vi "MeasLink Plugin Path.vi"(11 "error in (no error)":errorcluster) -> (0 "Measurement UI Lib":path, 1 "Run Service":path, 2 "Measurement UI":path, 3 "Instrumentstudio Folder":path, 4 "New Code Module":path, 5 "Set Default Value":path, 6 "Wrapper Path":path, 8 "Result Control":path, 10 "Input Controls":path, 12 "Library":path, 13 "Type Specialization":path, 14 "Logic VI Path":path, 15 "error out":errorcluster)   [LabVIEW 2021, in "Path Functions.lvlib"]
uses:
  Path Functions.lvlib
  Converter Reusables/Converter Reusables.lvlib
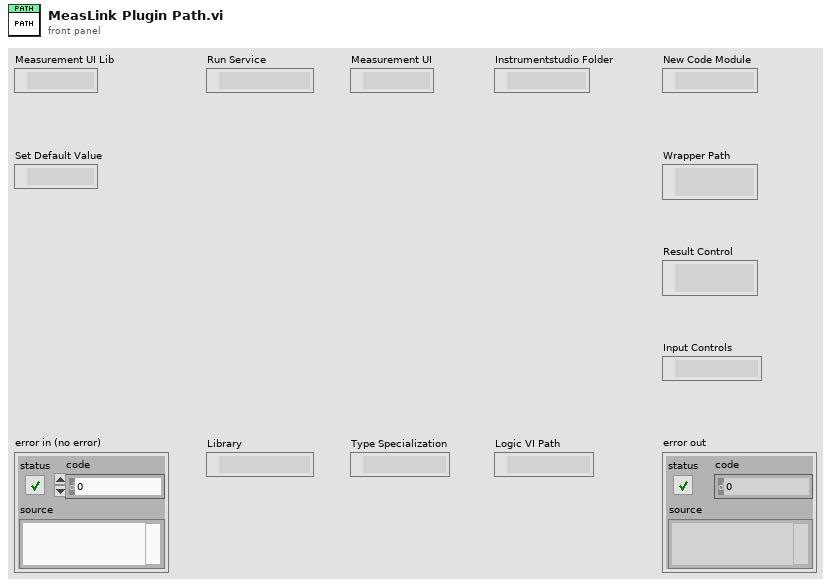
[diagram p1: front panel]
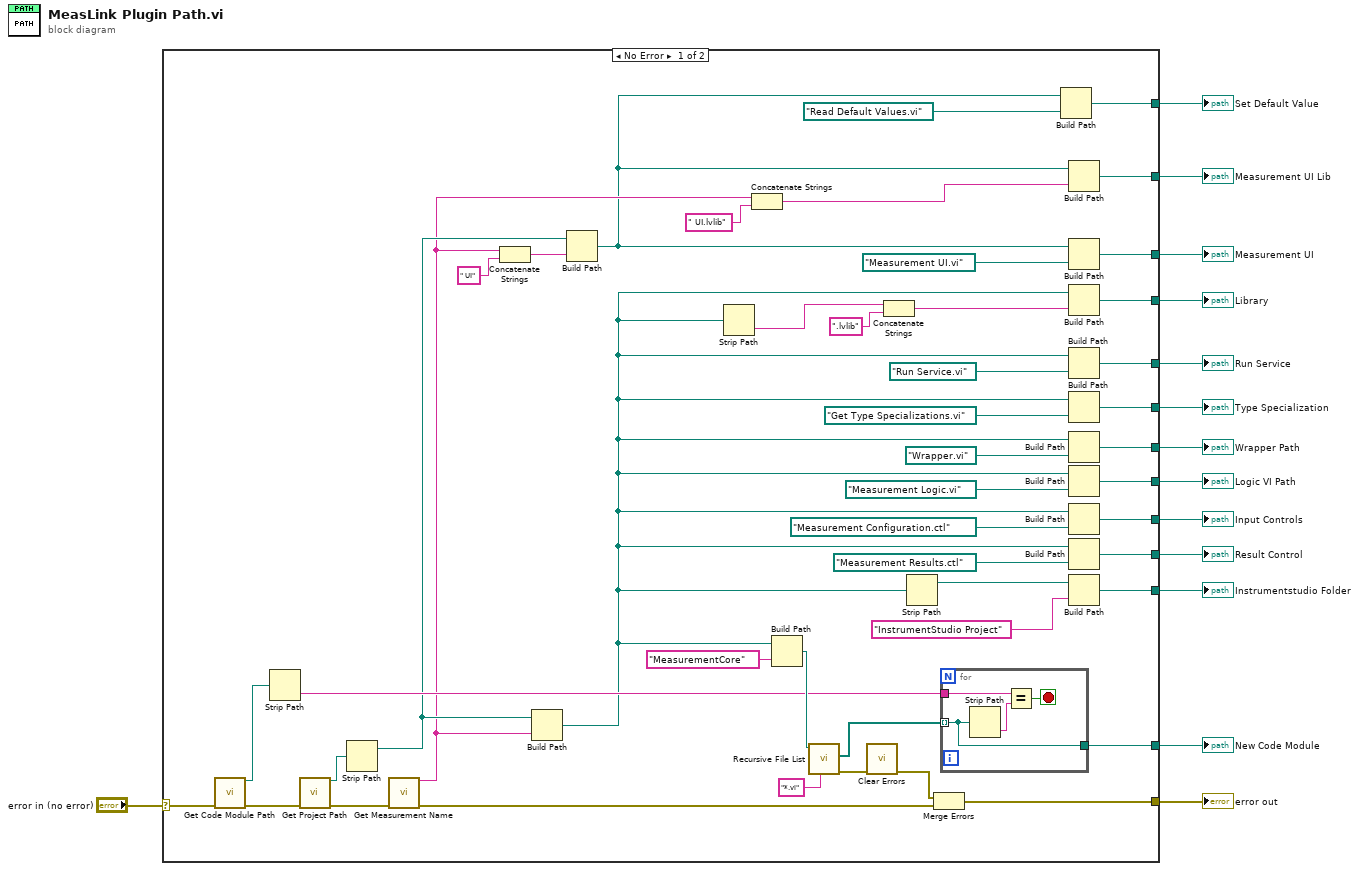
[diagram p0: block diagram]
diagram:
  n1 = case shown="No Error" "error in (no error)" {
    selector: "error in (no error)" -> [w42 w66]
    tunnel: [w61 _] -> w14
    tunnel: [w60 _] -> w13
    tunnel: [w59 _] -> w12
    tunnel: [w58 _] -> w11
    tunnel: [w52 _] -> w10
    tunnel: [w51 _] -> w9
    tunnel: [w49 _] -> w8
    tunnel: [w45 _] -> w7
    tunnel: [w38 _] -> w5
    tunnel: [w27 w66] -> w4
    tunnel: [w26 _] -> w3
    tunnel: [w18 _] -> w2
    tunnel: [w17 _] -> w1
    frame No Error {
      n2 = call "Get Code Module Path.vi"("error in (no error)"=w42) -> ("CodeModule Out"=w40:path, "error out"=w41:errorcluster)  [unwired: 13 in]
      n3 = Strip Path(path=w40) -> (name=w29:string)  [unwired: 1 out]
      n4 = call "Get Project Path.vi"("error in (no error)"=w41) -> ("Project Path Out"=w44:path, "error out"=w43:errorcluster)  [unwired: 13 in]
      n5 = Strip Path(path=w44) -> (stripped path=w24:path)  [unwired: 1 out]
      n6 = call "Get Measurement Name.vi"("error in (no error)"=w43) -> ("Name Out"=w19:string, "error out"=w28:errorcluster)  [unwired: 13 in]
      n7 = Concatenate Strings(w19, " UI" ("string")) -> (w22:string)
      n8 = Build Path(base path=w24, name or relative path=w19) -> (appended path=w25:path)
      n9 = Build Path(base path=w24, name or relative path=w22) -> (appended path=w16:path)
      n10 = Strip Path(path=w25) -> (name=w39:string)  [unwired: 1 out]
      n11 = Concatenate Strings(w19, " UI.lvlib" ("string")) -> (w20:string)
      n12 = Build Path(base path=w25, name or relative path="MeasurementCore" ("string")) -> (appended path=w32:path)
      n13 = call <vilib>:"Recursive File List.vi"("pattern"="*.vi", "Folder Path"=w32) -> ("error out"=w31:errorcluster, "All Files in Dir"=w33:path[])  [unwired: 5 in, 3 out]
      n14 = call <vilib>:"Clear Errors.vi"("error in (no error)"=w31) -> ("error out"=w30:errorcluster)  [unwired: 5 in, 1 out]
      n15 = Concatenate Strings(w39, ".lvlib" ("string")) -> (w37:string)
      n16 = Strip Path(path=w25) -> (stripped path=w48:path)  [unwired: 1 out]
      n17 = Merge Errors(w30, w28) -> (w27:errorcluster)
      n18 = for {
        tunnel: w33 -> [w63] mode=indexing
        tunnel: w29 -> [w65]
        tunnel: [w63] -> w26
        stop <- w62 stop-if-true
        n19 = Strip Path(path=w63) -> (name=w64:string)  [unwired: 1 out]
        n20 = Equal?(x=w65, y=w64) -> (x = y?=w62:bool)
      }
      n21 = Build Path(base path=w16, name or relative path=path "Read Default Values.vi") -> (appended path=w17:path)
      n22 = Build Path(base path=w16, name or relative path=w20) -> (appended path=w18:path)
      n23 = Build Path(base path=w16, name or relative path=path "Measurement UI.vi") -> (appended path=w52:path)
      n24 = Build Path(base path=w25, name or relative path=w37) -> (appended path=w38:path)
      n25 = Build Path(base path=w25, name or relative path=path "Run Service.vi") -> (appended path=w45:path)
      n26 = Build Path(base path=w25, name or relative path=path "Get Type Specializations.vi") -> (appended path=w51:path)
      n27 = Build Path(base path=w25, name or relative path=path "Wrapper.vi") -> (appended path=w61:path)
      n28 = Build Path(base path=w25, name or relative path=path "Measurement Logic.vi") -> (appended path=w60:path)
      n29 = Build Path(base path=w25, name or relative path=path "Measurement Configuration.ctl") -> (appended path=w59:path)
      n30 = Build Path(base path=w25, name or relative path=path "Measurement Results.ctl") -> (appended path=w58:path)
      n31 = Build Path(base path=w48, name or relative path="InstrumentStudio Project" ("string")) -> (appended path=w49:path)
    }
    frame Error {
    }
  }
  "error out" <- w4
  "New Code Module" <- w3
  "Wrapper Path" <- w14
  "Logic VI Path" <- w13
  "Input Controls" <- w12
  "Result Control" <- w11
  "Instrumentstudio Folder" <- w8
  "Measurement UI" <- w10
  "Type Specialization" <- w9
  "Run Service" <- w7
  "Library" <- w5
  "Measurement UI Lib" <- w2
  "Set Default Value" <- w1
